vi "vision angle pid.vi"(0 "Mode":T1(ring), 1 "angle PID gains":T2={"proportional gain (Kc)"=1.0, "integral time (Ti, min)"=0.01, "derivative time (Td, min)"=0.0}, 2 "distance PID gains":T2={"proportional gain (Kc)"=1.0, "integral time (Ti, min)"=0.01, "derivative time (Td, min)"=0.0}, 5 "current angle":dbl, 9 "set distance":dbl, 11 "current distance":dbl, 12 "output range":cluster{"output high":dbl, "output low":dbl}={"output high"=100.0, "output low"=-100.0} {"output low" format="%.2f"; "output high" format="%.2f"}) -> (4 "left velocity":dbl format="%.2f", 6 "right velocity":dbl format="%.2f")   [LabVIEW 2020]
uses:
  <vilib>/addons/control/pid/pid.llb/PID (DBL).vi
  <vilib>/addons/control/pid/NI_PID_pid.lvlib
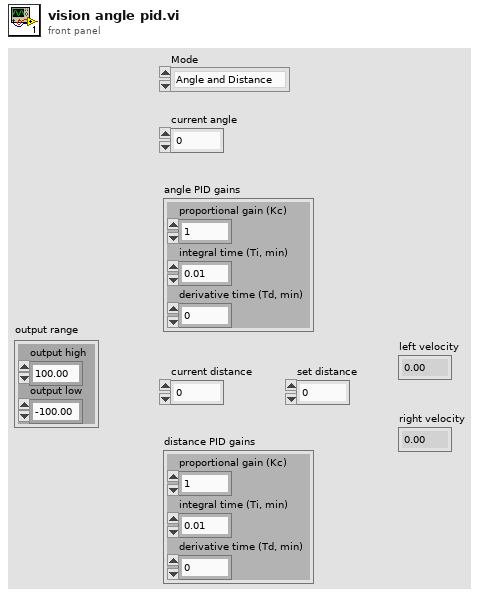
[diagram p1: front panel]
types:
  T1 = enum16{"Angle and Distance", "Distance", "Angle"}
  T2 = cluster{"proportional gain (Kc)":dbl, "integral time (Ti, min)":dbl, "derivative time (Td, min)":dbl}
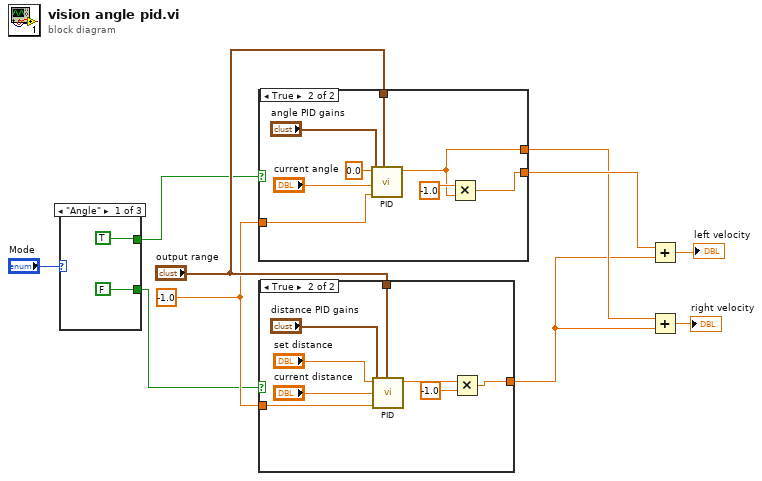
[diagram p0: block diagram]
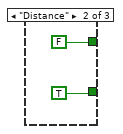
[diagram p2: hidden frame]
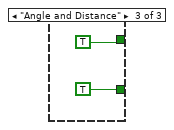
[diagram p3: hidden frame]
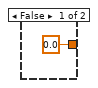
[diagram p4: hidden frame]
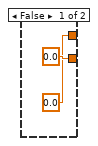
[diagram p5: hidden frame]
diagram:
  w5 = -1.0 ("dt (s)")
  n1 = case shown="\"Angle\"" "Mode" {
    tunnel: [TRUE FALSE TRUE] -> w2
    tunnel: [FALSE TRUE TRUE] -> w1
    frame "Angle" {
    }
    frame "Distance" {
    }
    frame "Angle and Distance" {
    }
  }
  n2 = case shown="True" w2 {
    tunnel: [0.0 ("output") w20] -> w9
    tunnel: [0.0 w19] -> w7
    tunnel: "output range" -> [_ w23]
    tunnel: w5 -> [_ w22]
    frame False {
    }
    frame True {
      n3 = call-poly <vilib>:"PID.vi"("output range"=w23, "dt (s)"=w22, "PID gains"="angle PID gains", "process variable"="current angle", "setpoint"=0.0) -> ("output"=w19:dbl)  [unwired: 5 in, 1 out]
      n4 = Multiply(x=-1.0, y=w19) -> (x*y=w20:dbl)
    }
  }
  n5 = case shown="True" w1 {
    tunnel: [0.0 ("output") w29] -> w4
    tunnel: "output range" -> [_ w33]
    tunnel: w5 -> [_ w32]
    frame False {
    }
    frame True {
      n6 = call-poly <vilib>:"PID.vi"("output range"=w33, "dt (s)"=w32, "PID gains"="distance PID gains", "process variable"="current distance", "setpoint"="set distance") -> ("output"=w30:dbl)  [unwired: 5 in, 1 out]
      n7 = Multiply(x=w30, y=-1.0) -> (x*y=w29:dbl)
    }
  }
  n8 = Add(x=w9, y=w4) -> (x+y=→"left velocity":dbl)
  n9 = Add(x=w7, y=w4) -> (x+y=→"right velocity":dbl)
